vi "2013_01_24 Flow Main.vi"() -> ()   [LabVIEW 2013]
uses:
  Flow Type Def.ctl
  flow and pressure.ctl
  <vilib>/DAQmx/write.llb/DAQmx Write (Counter Time 1Chan 1Samp).vi
  <vilib>/DAQmx/read.llb/DAQmx Read (Analog 1D Wfm NChan NSamp).vi
  <vilib>/DAQmx/miscellaneous.llb/DAQmx Fill In Error Info.vi
  <resource>/objmgr/daqmx.rc
panel:
  in  "Zero":bool
  in  "Clear":bool
  out "TotalSampPerChanAcquired":dbl
  out "AvailSampPerChan":u32
  out "XY Graph 3":cluster{"Array":dbl[], "Array":dbl[]}[](graph)
  in  "Flow Loop":T1 {"Thermometer" scale=15.0..50.0; "Pressure Up (mmHg)" format="%#.1g"; "Pressure Down (mmHg)" format="%#.1g"; "Zero Up" format="%.2f"; "Hydraulic Power" scale=0.0..0.1 scale format="%#.2f"; "Flow" scale=0.0..8.0 scale format="%#.2f"; "Pressure Difference" scale=0.0..10.0 scale format="%#.2f"}
  in  "Y axis":u16(ring)=3 items=["RMS Current (A) 1"=1, "RMS Voltage (V) 1"=2, "RPM"=3, "Supply (V)"=4, "Torque (mNm)"=5, "Electrical Power (W)"=6, "Mechanical Power(W)"=7, "Motor Efficiency (%)"=8, "Source Current (A)"=10, "Supply Power (W)"=11, "ESC Efficiency (%)"=12, "Flow"=13, "Pressure Blue"=14, "Pressure Yellow"=15, "etc"=16]
  in  "X axis":u16(ring)=5 items=["RMS Current (A) 1"=1, "RMS Voltage (V) 1"=2, "RPM"=3, "Supply (V)"=4, "Torque (mNm)"=5, "Electrical Power (W)"=6, "Mechanical Power(W)"=7, "Motor Efficiency (%)"=8, "Source Current (A)"=10, "Supply Power (W)"=11, "ESC Efficiency (%)"=12, "Flow"=13, "Pressure Blue"=14, "Pressure Yellow"=15, "etc"=16]
  in  "Write Comment":bool
  in  "Save":bool
  in  "Comments":string
  in  "Test ID and Serial #s":string
  in  "Motor 2":T2={"Fail"=FALSE, "RPM"=0, "Motor"=enum."Maxon EC6 6V", "ESC"=enum."Phoenix 10", "Supply (V)"=0.0, "Elapsed Time"=0.0, "Counter"=0.0, "Torque (mNm)"=0.0, "Electrical Power (W)"=0.0, "Motor Efficiency"=0.0, "Mechanical Power (W)"=0.0, "Supply Power (W)"=0.0, "ESC Efficiency"=0.0, "PWM"=0, "Direction"=enum."Push"} {"PWM" min=0 max=100 step=1 scale=0.0..100.0; "ESC Efficiency" format="%#_3g%%"; "Supply Power (W)" format="%.3g"; "Mechanical Power (W)" format="%.3g"; "Motor Efficiency" format="%#_3g%%"; "Electrical Power (W)" format="%.3g"; "Torque (mNm)" format="%.3g"; "Elapsed Time" format="%<%H:%M:%S>t"; "Supply (V)" format="%.2f"; "RPM" scale=0.0..60000.0}
  out "XY Graph 2":cluster{"Array":dbl[], "Array":dbl[]}[](graph)
  out "XY Graph":cluster{"Array":dbl[], "Array":dbl[]}(graph)
  out "error out":errorcluster
  in  "File Path":path=path "C:/Users/FlowLoop/Desktop/LabVIEW Results/.csv"
  in  "Motor 1":T2={"Fail"=FALSE, "RPM"=0, "Motor"=enum."", "ESC"=enum."Phoenix 10", "Supply (V)"=0.0, "Elapsed Time"=0.0, "Counter"=0.0, "Torque (mNm)"=0.0, "Electrical Power (W)"=0.0, "Motor Efficiency"=0.0, "Mechanical Power (W)"=0.0, "Supply Power (W)"=0.0, "ESC Efficiency"=0.0, "PWM"=0, "Direction"=enum."Pull"} {"PWM" min=0 max=100 step=1 scale=0.0..100.0; "ESC Efficiency" format="%#_3g%%"; "Supply Power (W)" format="%.3g"; "Mechanical Power (W)" format="%.3g"; "Motor Efficiency" format="%#_3g%%"; "Electrical Power (W)" format="%.3g"; "Torque (mNm)" format="%.3g"; "Elapsed Time" format="%<%H:%M:%S>t"; "Supply (V)" format="%.2f"; "RPM" scale=0.0..60000.0}
  out "loop time (ms)":u32
  in  "stop":bool
  # "DEL to activate\nRETURN to write"
  # "1. Select Motor/ESC/Direction\n2. Give file descriptive name or 'test' if you don't want to keep data\n3. Hit record. Clear erases data and starts new file.\n4. Zero the pressure with 'Zero P' button.\n5. Run motor in air and mounted in can, make sure torque @12V <0.13\n6. Control Motor with WM slider.\n7. Enter comments by clicking in comments field or pressing DEL and typing. Write comment with ENTER or 'Write' button.\n8. Interact with graphs using visible plot selectors or x/y dropdowns.\n9. Files written to Desktop/Labview Results. Analyze with NI DIAdem scripts."
  # "notes for fluorescence:\nstart stop motor\nsingle particle\nparticle burst\ncontinuous particles\npan\nreverse direction if particles clogged"
  # "todo: \nwrite file fix\ncomments\nzero pressure"
  # "Stopped"
  # "Stopped"
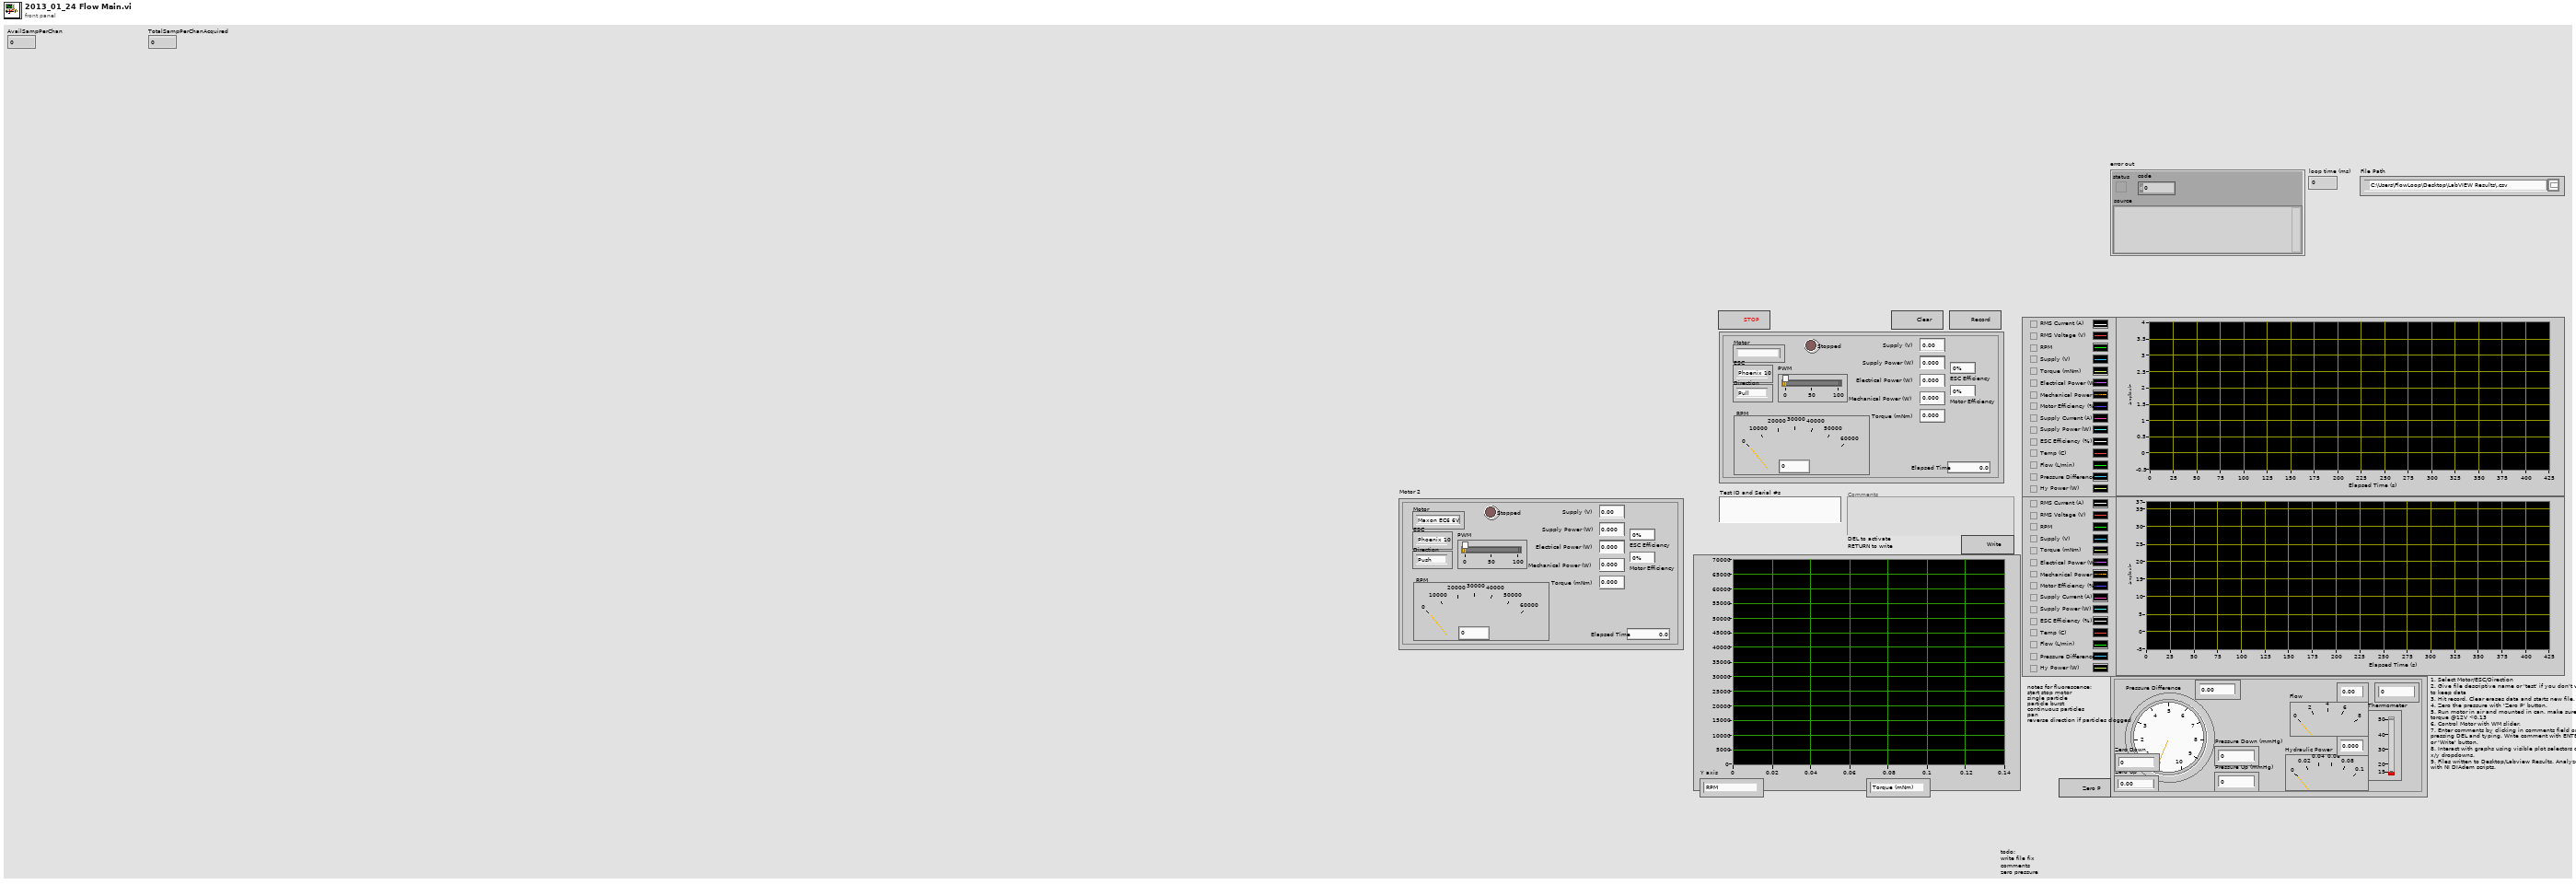
[diagram p1: front panel]
types:
  T1 = typedef "flow and pressure.ctl" = cluster{"Pressure Difference":dbl, "Flow":dbl, "Hydraulic Power":dbl, "Zero Up":dbl, "Pressure Down (mmHg)":dbl, "Pressure Up (mmHg)":dbl, "Zero Down":dbl, "Thermometer":dbl}
  T2 = typedef "Flow Type Def.ctl" = cluster{"Fail":bool, "RPM":u64, "Motor":enum16{"", "Maxon EC6 6V", "Maxon EC4 6V", "FH 0620 6V", "FH 0620 12V", "FH 0427"}, "ESC":enum16{"Phoenix 10", "Maxon", "FH 1801"}, "Supply (V)":dbl, "Elapsed Time":dbl, "Counter":dbl, "Torque (mNm)":dbl, "Electrical Power (W)":dbl, "Motor Efficiency":dbl, "Mechanical Power (W)":dbl, "Supply Power (W)":dbl, "ESC Efficiency":dbl, "PWM":i32, "Direction":enum16{"Push", "Pull"}}
  T3 = enum8{"Enabled", "Disabled", "Disabled and Grayed Out"}
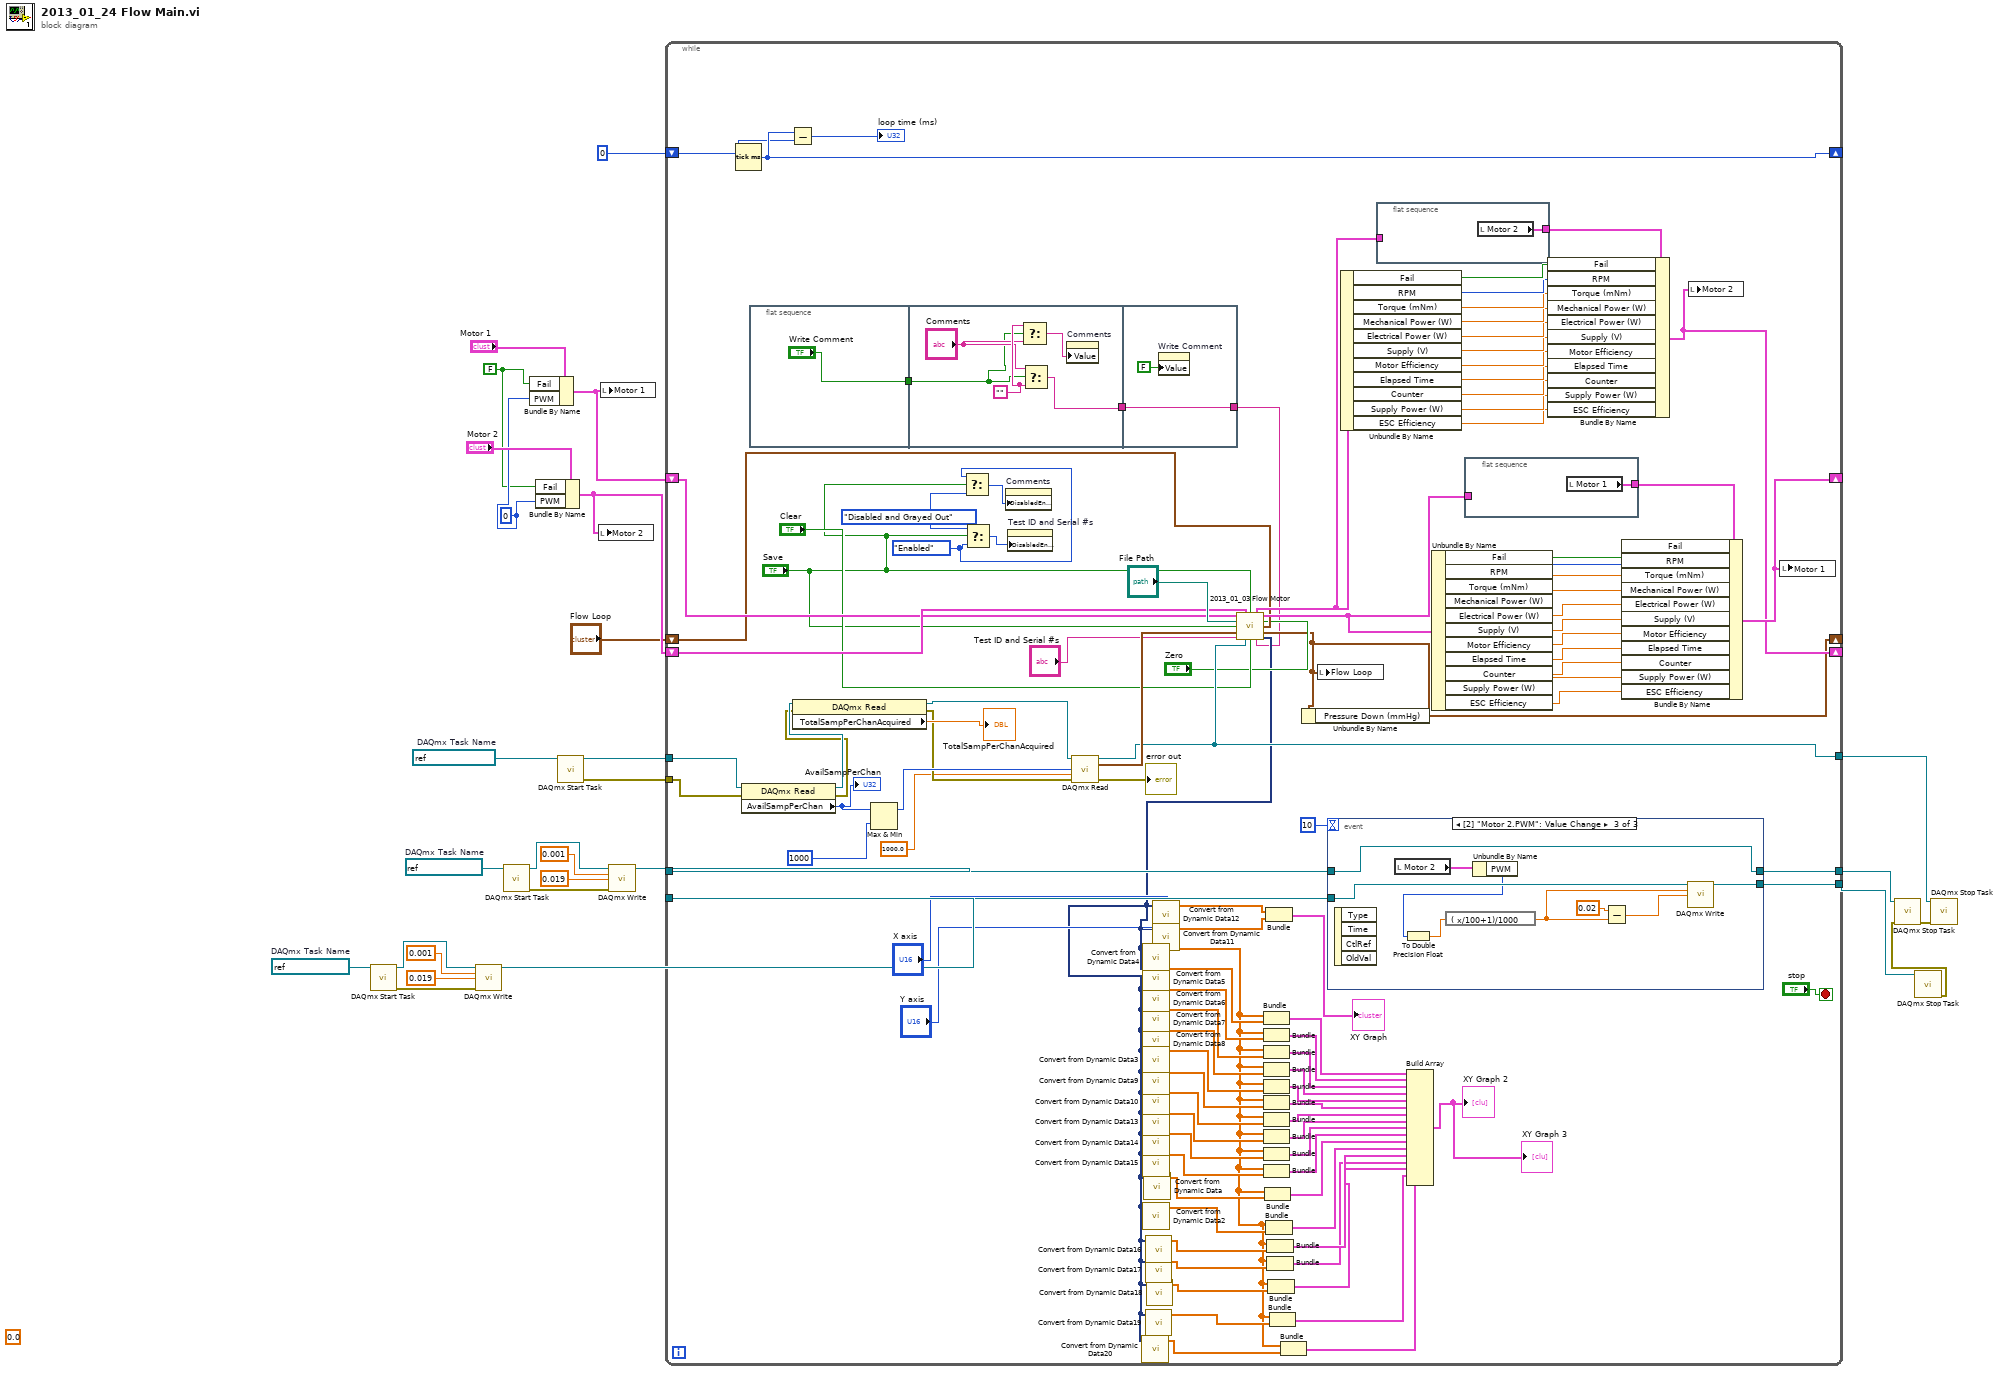
[diagram p0: block diagram]
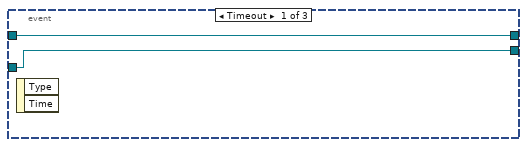
[diagram p2: hidden frame]
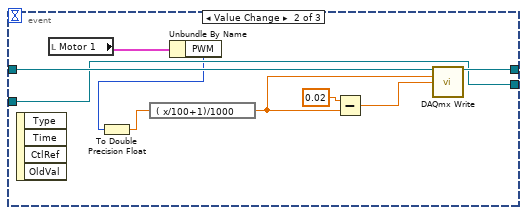
[diagram p3: hidden frame]
diagram:
  w3 = 0 ("PWM")
  w13 = refnum<k21> "Flow PWM2"  # DAQmx Task Name
  w2 = FALSE ("Enabled")
  (unwired) 0.0 ("PWM 1")
  w25 = refnum<k21> "Flow PWM1"  # DAQmx Task Name
  w28 = refnum<k21> "Flow Acquire"  # DAQmx Task Name
  n1 = call <vilib>:"DAQmx Start Task.vi"("task/channels in"=w13) -> ("task out"=w12:refnum<k21>, "error out"=w11:errorcluster)  [unwired: 13 in]
  n2 = call-poly <vilib>:"DAQmx Write.vi"("task/channels in"=w12, "high time"=0.001 ("data"), "low time"=0.019 ("data"), "error in"=w11) -> ("task out"=w8:refnum<k21>)  [unwired: 9 in, 2 out]
  n3 = call <vilib>:"DAQmx Start Task.vi"("task/channels in"=w25) -> ("task out"=w23:refnum<k21>, "error out"=w22:errorcluster)  [unwired: 13 in]
  n4 = Bundle By Name(cluster="Motor 1", "Fail"=w2, "PWM"=w3) -> (w14:T2)
  n5 = Bundle By Name(cluster="Motor 2", "Fail"=w2, "PWM"=w3) -> (w4:T2)
  n6 = call <vilib>:"DAQmx Start Task.vi"("task/channels in"=w28) -> ("task out"=w27:refnum<k21>, "error out"=w16:errorcluster)  [unwired: 13 in]
  n7 = local write "Motor 2"(w4) -> ()
  n8 = local write "Motor 1"(w14) -> ()
  n9 = call-poly <vilib>:"DAQmx Write.vi"("task/channels in"=w23, "high time"=0.001 ("data"), "low time"=0.019 ("data"), "error in"=w22) -> ("task out"=w24:refnum<k21>)  [unwired: 9 in, 2 out]
  n10 = while {
    tunnel: w27 -> [w48]
    tunnel: [w56] -> w26
    tunnel: w16 -> [w49]
    shift-right: [w136] -> _
    shift-left: u32 0 ("millisecond timer value") -> [w135]
    tunnel: w24 -> [w133]
    tunnel: [w58] -> w21
    shift-right: [w121] -> _
    shift-left: w14 -> [w43]
    tunnel: w8 -> [w92]
    tunnel: [w91] -> w7
    shift-right: [w76] -> _
    shift-left: w4 -> [w44]
    shift-right: [w34] -> _
    shift-left: "Flow Loop" -> [w37]
    stop <- "stop" stop-if-true
    w39 = T3."Enabled" ("Disabled")
    w40 = T3."Disabled and Grayed Out" ("Disabled")
    n11 = Tick Count (ms)() -> (millisecond timer value=w136:u32)
    n12 = property class="DAQmx Read"(reference=w48, error in=w49) -> (reference out=w55:refnum<k21>, error out=w54:errorcluster, "AvailSampPerChan"=w53:u32)
    "AvailSampPerChan" <- w53
    n13 = flat-sequence {
      tunnel: ["Write Comment"] -> w59
      tunnel: [w139] -> w60
      tunnel: w59 -> [w140]
      tunnel: [w145] -> w29
      tunnel: w60 -> [w145]
      frame #0 {
      }
      frame #1 {
        w143 = ""
        n14 = Select(t=w143, s=w140, f="Comments") -> (s? t:f=w142:string)
        n15 = Select(t="Comments", s=w140, f=w143) -> (s? t:f=w139:string)
        n16 = property on="Comments" class="Str"("Value"=w142) -> ()  [unwired: 2 in, 2 out]
      }
      frame #2 {
        n17 = property on="Write Comment" class="Bool (strict)"("Value"=FALSE ("Save Button")) -> ()  [unwired: 2 in, 2 out]
      }
    }
    n18 = Subtract(x=w136, y=w135) -> (x-y=→"loop time (ms)":u32)
    n19 = property class="DAQmx Read"(reference=w55, error in=w54) -> (reference out=w47:refnum<k21>, error out=w46:errorcluster, "TotalSampPerChanAcquired"=→"TotalSampPerChanAcquired":dbl)
    n20 = Max & Min(x=w53, y=1000 ("number of samples per channel")) -> (max(x,y)=w50:u32)  [unwired: 1 out]
    n21 = Select(t=w39, s="Save", f=w40) -> (s? t:f=w38:T3)
    n22 = Select(t=w40, s="Save", f=w39) -> (s? t:f=w41:T3)
    n23 = property on="Comments" class="Str"("DisabledEnum"=w38) -> ()  [unwired: 2 in, 2 out]
    n24 = property on="Test ID and Serial #s" class="Str"("DisabledEnum"=w41) -> ()  [unwired: 2 in, 2 out]
    n25 = call-poly <vilib>:"DAQmx Read.vi"("task/channels in"=w47, "number of samples per channel"=w50, "timeout"=1000.0, "error in"=w46) -> ("task out"=w56:refnum<k21>, "data"=w74:waveform(dbl)[], "error out"=→"error out":errorcluster)  [unwired: 9 in]
    n26 = call "2013_01_03 Flow Motor.vi"("Motor Typedef"=w43, "Motor Typedef 2"=w44, "Capture"="Save", "File Path"="File Path", "Zero"="Zero", "Save"="Save", "Flow in"=w37, "data"=w74, "File ID and Serial #s"="Test ID and Serial #s", "DAQmx Task Name"=w56, "Clear"="Clear", "Comment"=w29) -> ("Motor Typedef Out 2"=w72:T2, "Motor Typedef Out"=w120:T2, "Flow and P out"=w34:T1, "Final Out"=w33:dynamicdata)
    n27 = call "Convert from Dynamic Data20"("Dynamic Data Type"=w33) -> ("Array"=w31:dbl[])  [unwired: 3 in]
    n28 = call "Convert from Dynamic Data4"("Dynamic Data Type"=w33) -> ("Array"=w32:dbl[])  [unwired: 3 in]
    n29 = call "Convert from Dynamic Data5"("Dynamic Data Type"=w33) -> ("Array"=w109:dbl[])  [unwired: 3 in]
    n30 = call "Convert from Dynamic Data6"("Dynamic Data Type"=w33) -> ("Array"=w108:dbl[])  [unwired: 3 in]
    n31 = call "Convert from Dynamic Data7"("Dynamic Data Type"=w33) -> ("Array"=w107:dbl[])  [unwired: 3 in]
    n32 = call "Convert from Dynamic Data8"("Dynamic Data Type"=w33) -> ("Array"=w106:dbl[])  [unwired: 3 in]
    n33 = call "Convert from Dynamic Data3"("Dynamic Data Type"=w33) -> ("Array"=w105:dbl[])  [unwired: 3 in]
    n34 = call "Convert from Dynamic Data9"("Dynamic Data Type"=w33) -> ("Array"=w104:dbl[])  [unwired: 3 in]
    n35 = call "Convert from Dynamic Data10"("Dynamic Data Type"=w33) -> ("Array"=w103:dbl[])  [unwired: 3 in]
    n36 = call "Convert from Dynamic Data13"("Dynamic Data Type"=w33) -> ("Array"=w102:dbl[])  [unwired: 3 in]
    n37 = call "Convert from Dynamic Data14"("Dynamic Data Type"=w33) -> ("Array"=w101:dbl[])  [unwired: 3 in]
    n38 = call "Convert from Dynamic Data15"("Dynamic Data Type"=w33) -> ("Array"=w100:dbl[])  [unwired: 3 in]
    n39 = call "Convert from Dynamic Data2"("Dynamic Data Type"=w33) -> ("Array"=w97:dbl[])  [unwired: 3 in]
    n40 = call "Convert from Dynamic Data"("Dynamic Data Type"=w33) -> ("Array"=w99:dbl[])  [unwired: 3 in]
    n41 = call "Convert from Dynamic Data16"("Dynamic Data Type"=w33) -> ("Array"=w68:dbl[])  [unwired: 3 in]
    n42 = call "Convert from Dynamic Data17"("Dynamic Data Type"=w33) -> ("Array"=w67:dbl[])  [unwired: 3 in]
    n43 = call "Convert from Dynamic Data19"("Dynamic Data Type"=w33) -> ("Array"=w65:dbl[])  [unwired: 3 in]
    n44 = call "Convert from Dynamic Data18"("Dynamic Data Type"=w33) -> ("Array"=w66:dbl[])  [unwired: 3 in]
    n45 = call "Convert from Dynamic Data12"("Dynamic Data Type"=w33, "Channel"="X axis") -> ("Array"=w89:dbl[])  [unwired: 2 in]
    n46 = call "Convert from Dynamic Data11"("Dynamic Data Type"=w33, "Channel"="Y axis") -> ("Array"=w90:dbl[])  [unwired: 2 in]
    n47 = Bundle("Array"=w32, "Array"=w109) -> (w110:cluster{"Array":dbl[], "Array":dbl[]})  [unwired: 1 in]
    n48 = Bundle("Array"=w32, "Array"=w108) -> (w111:cluster{"Array":dbl[], "Array":dbl[]})  [unwired: 1 in]
    n49 = Bundle("Array"=w32, "Array"=w107) -> (w112:cluster{"Array":dbl[], "Array":dbl[]})  [unwired: 1 in]
    n50 = Bundle("Array"=w32, "Array"=w106) -> (w113:cluster{"Array":dbl[], "Array":dbl[]})  [unwired: 1 in]
    n51 = Bundle("Array"=w32, "Array"=w105) -> (w114:cluster{"Array":dbl[], "Array":dbl[]})  [unwired: 1 in]
    n52 = Bundle("Array"=w32, "Array"=w104) -> (w115:cluster{"Array":dbl[], "Array":dbl[]})  [unwired: 1 in]
    n53 = Bundle("Array"=w32, "Array"=w103) -> (w116:cluster{"Array":dbl[], "Array":dbl[]})  [unwired: 1 in]
    n54 = Bundle("Array"=w32, "Array"=w102) -> (w117:cluster{"Array":dbl[], "Array":dbl[]})  [unwired: 1 in]
    n55 = Bundle("Array"=w32, "Array"=w101) -> (w119:cluster{"Array":dbl[], "Array":dbl[]})  [unwired: 1 in]
    n56 = Bundle("Array"=w32, "Array"=w100) -> (w118:cluster{"Array":dbl[], "Array":dbl[]})  [unwired: 1 in]
    n57 = Bundle("Array"=w32, "Array"=w99) -> (w98:cluster{"Array":dbl[], "Array":dbl[]})  [unwired: 1 in]
    n58 = Bundle("Array"=w89, "Array"=w90) -> (→"XY Graph":cluster{"Array":dbl[], "Array":dbl[]})  [unwired: 1 in]
    n59 = Bundle("Array"=w32, "Array"=w97) -> (w96:cluster{"Array":dbl[], "Array":dbl[]})  [unwired: 1 in]
    n60 = Bundle("Array"=w32, "Array"=w68) -> (w64:cluster{"Array":dbl[], "Array":dbl[]})  [unwired: 1 in]
    n61 = Bundle("Array"=w32, "Array"=w67) -> (w63:cluster{"Array":dbl[], "Array":dbl[]})  [unwired: 1 in]
    n62 = Bundle("Array"=w32, "Array"=w66) -> (w62:cluster{"Array":dbl[], "Array":dbl[]})  [unwired: 1 in]
    n63 = Bundle("Array"=w32, "Array"=w65) -> (w61:cluster{"Array":dbl[], "Array":dbl[]})  [unwired: 1 in]
    n64 = Bundle("Array"=w32, "Array"=w31) -> (w30:cluster{"Array":dbl[], "Array":dbl[]})  [unwired: 1 in]
    n65 = Unbundle By Name(w34) -> ()  [unwired: 1 out]
    n66 = local write "Flow Loop"(w34) -> ()
    n67 = event shown="[2] \"Motor 2.PWM\": Value Change" {
      selector: _ -> [_ _ _]
      dyn-events: _ -> [_ _ _]
      timeout: 10 -> [_ _ _]
      tunnel: w133 -> [w149 w155 w162]
      tunnel: [w149 w154 w162] -> w58
      tunnel: w92 -> [w148 w153 w164]
      tunnel: [w148 w153 w163] -> w91
      event Timeout {
        n68 = event-data() -> ()  [unwired: 1 in, 2 out]
      }
      event Value Change {
        n69 = event-data() -> ()  [unwired: 1 in, 4 out]
        n70 = local read "Motor 1"() -> (w151:T2)
        n71 = Unbundle By Name(w151) -> ("PWM"=w150:i32)
        n72 = To Double Precision Float(number=w150) -> (double precision float=w152:dbl)
        n73 = expression code="( x/100+1)/1000"(w152) -> (w156:dbl)
        n74 = Subtract(x=0.02 ("y"), y=w156) -> (x-y=w157:dbl)
        n75 = call-poly <vilib>:"DAQmx Write.vi"("task/channels in"=w155, "high time"=w156, "low time"=w157) -> ("task out"=w154:refnum<k21>)  [unwired: 10 in, 2 out]
      }
      event Value Change {
        n76 = event-data() -> ()  [unwired: 1 in, 4 out]
        n77 = local read "Motor 2"() -> (w160:T2)
        n78 = Unbundle By Name(w160) -> ("PWM"=w159:i32)
        n79 = To Double Precision Float(number=w159) -> (double precision float=w161:dbl)
        n80 = expression code="( x/100+1)/1000"(w161) -> (w165:dbl)
        n81 = Subtract(x=0.02 ("y"), y=w165) -> (x-y=w166:dbl)
        n82 = call-poly <vilib>:"DAQmx Write.vi"("task/channels in"=w164, "high time"=w165, "low time"=w166) -> ("task out"=w163:refnum<k21>)  [unwired: 10 in, 2 out]
      }
    }
    n83 = Unbundle By Name(w72) -> ("Fail"=w87:bool, "RPM"=w86:u64, "Torque (mNm)"=w85:dbl, "Mechanical Power (W)"=w84:dbl, "Electrical Power (W)"=w83:dbl, "Supply (V)"=w82:dbl, "Motor Efficiency"=w81:dbl, "Elapsed Time"=w80:dbl, "Counter"=w79:dbl, "Supply Power (W)"=w78:dbl, "ESC Efficiency"=w77:dbl)
    n84 = flat-sequence {
      tunnel: [w146] -> w75
      tunnel: w72 -> [_]
      frame #0 {
        n85 = local read "Motor 2"() -> (w146:T2)
      }
    }
    n86 = Build Array(w110, w111, w112, w113, w114, w115, w116, w117, w119, w118, w98, w96, w64, w63, w62, w61, w30) -> (→"XY Graph 2" →"XY Graph 3":cluster{"Array":dbl[], "Array":dbl[]}[])
    n87 = Unbundle By Name(w120) -> ("Fail"=w130:bool, "RPM"=w129:u64, "Torque (mNm)"=w128:dbl, "Mechanical Power (W)"=w127:dbl, "Electrical Power (W)"=w126:dbl, "Supply (V)"=w125:dbl, "Motor Efficiency"=w124:dbl, "Elapsed Time"=w123:dbl, "Counter"=w122:dbl, "Supply Power (W)"=w94:dbl, "ESC Efficiency"=w95:dbl)
    n88 = flat-sequence {
      tunnel: w120 -> [_]
      tunnel: [w147] -> w93
      frame #0 {
        n89 = local read "Motor 1"() -> (w147:T2)
      }
    }
    n90 = Bundle By Name(cluster=w75, "Fail"=w87, "RPM"=w86, "Torque (mNm)"=w85, "Mechanical Power (W)"=w84, "Electrical Power (W)"=w83, "Supply (V)"=w82, "Motor Efficiency"=w81, "Elapsed Time"=w80, "Counter"=w79, "Supply Power (W)"=w78, "ESC Efficiency"=w77) -> (w76:T2)
    n91 = Bundle By Name(cluster=w93, "Fail"=w130, "RPM"=w129, "Torque (mNm)"=w128, "Mechanical Power (W)"=w127, "Electrical Power (W)"=w126, "Supply (V)"=w125, "Motor Efficiency"=w124, "Elapsed Time"=w123, "Counter"=w122, "Supply Power (W)"=w94, "ESC Efficiency"=w95) -> (w121:T2)
    n92 = local write "Motor 2"(w76) -> ()
    n93 = local write "Motor 1"(w121) -> ()
  }
  n94 = call <vilib>:"DAQmx Stop Task.vi"("task/channels in"=w7) -> ("error out"=w6:errorcluster)  [unwired: 13 in, 1 out]
  n95 = call <vilib>:"DAQmx Stop Task.vi"("task/channels in"=w21, "error in"=w6) -> ("error out"=w20:errorcluster)  [unwired: 12 in, 1 out]
  n96 = call <vilib>:"DAQmx Stop Task.vi"("task/channels in"=w26, "error in"=w20) -> ()  [unwired: 12 in, 2 out]
